vi "Idle.vi"(8 "error in":errorcluster, 11 "Plugin_Driver in":refnum<class "Plugin_Driver.lvclass">) -> (0 "error out":errorcluster, 3 "Plugin_Driver out":refnum<class "Plugin_Driver.lvclass">)   [LabVIEW 2020, in "Plugin.lvlib" / "Plugin_Driver.lvclass"]
doc: "This VI is a wrapper API for Instrument Driver's Idle API"
uses:
  Plugin_Driver.lvclass
  Drivers/Instrument Driver/Instrument Driver.lvclass
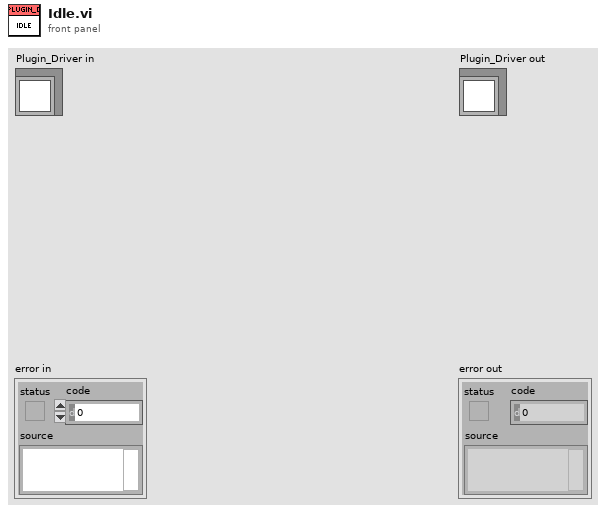
[diagram p1: front panel]
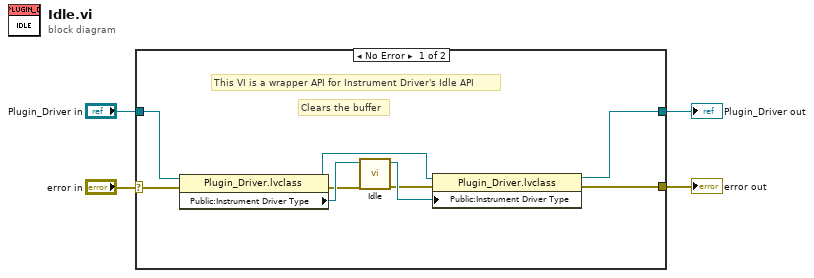
[diagram p0: block diagram]
diagram:
  n1 = case shown="No Error" "error in" {
    selector: "error in" -> [w8 w15]
    tunnel: [w7 w15] -> w3
    tunnel: [w5 w14] -> w1
    tunnel: "Plugin_Driver in" -> [w6 w14]
    frame No Error {
      # "This VI is a wrapper API for Instrument Driver's Idle API"
      # "Clears the buffer"
      n2 = property class="Plugin_Driver.lvclass"(reference=w6, error in=w8) -> (reference out=w12:refnum<class "Plugin_Driver.lvclass">, error out=w10:errorcluster, "Public:Instrument Driver Type"=w13:refnum<class "Instrument Driver.lvclass">)
      n3 = call-dynamic "Idle.vi"("error in (no error)"=w10, "Instrument Driver in"=w13) -> ("error out"=w9:errorcluster, "Instrument Driver out"=w11:refnum<class "Instrument Driver.lvclass">)  [unwired: 8 in]
      n4 = property class="Plugin_Driver.lvclass"(reference=w12, error in=w9, "Public:Instrument Driver Type"=w11) -> (reference out=w5:refnum<class "Plugin_Driver.lvclass">, error out=w7:errorcluster)
    }
    frame Error {
    }
  }
  "error out" <- w3
  "Plugin_Driver out" <- w1
